vi "Update_Data.vi"(8 "error in (no error)":errorcluster caption="entrée d'erreur (pas d'erreur)", 11 "Firebase Benches en entrée":refnum<class "Firebase Benches.lvclass">) -> (0 "error out":errorcluster caption="sortie d'erreur", 3 "Firebase Benches en sortie":refnum<class "Firebase Benches.lvclass">)   [LabVIEW 2020, in "Library Instrument & Equipement.lvlib" / "Library FireBase.lvlib" / "Firebase Benches.lvclass"]
doc: "Create New document\nPlease initialise the following values\n - Name BDD\n - Document\n - API Key"
uses:
  Firebase Benches.lvclass
  C:/Users/ngarcin/OneDrive - Altyor/Standard TB/Class/Firebase/Source/Firebase Driver/Firebase Driver.lvclass
  Firebase Benches.lvclass/Firebase Benches.ctl
  Firebase Altyor/Firebase Altyor.lvclass
  Firebase Driver/Firebase Driver.lvclass
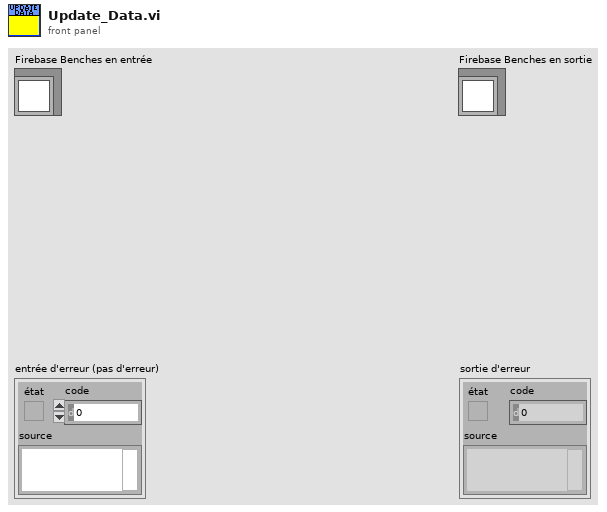
[diagram p1: front panel]
types:
  T1 = cluster{"fields":cluster{"Result":cluster{"booleanValue":bool}, "CreationDate":cluster{"timestampValue":string}, "Batch":cluster{"stringValue":string}, "SerialNumber":cluster{"stringValue":string}, "EndOfProduction":cluster{"timestampValue":string}, "FW_Version":cluster{"mapValue":cluster{"fields":cluster{"Bootloader":cluster{"mapValue":cluster{"fields":cluster{"File_Name":cluster{"stringValue":string}, "Version":cluster{"mapValue":cluster{"fields":cluster{"Major":cluster{"stringValue":string}, "Minor":cluster{"stringValue":string}}}}, "Checksum":cluster{"stringValue":string}}}}, "SoftDevice":cluster{"mapValue":cluster{"fields":cluster{"File_Name":cluster{"stringValue":string}, "Version":cluster{"mapValue":cluster{"fields":cluster{"Major":cluster{"stringValue":string}, "Minor":cluster{"stringValue":string}}}}, "Checksum":cluster{"stringValue":string}}}}, "DFU":cluster{"mapValue":cluster{"fields":cluster{"File_Name":cluster{"stringValue":string}, "Version":cluster{"mapValue":cluster{"fields":cluster{"Major":cluster{"stringValue":string}, "Minor":cluster{"stringValue":string}}}}, "Checksum":cluster{"stringValue":string}}}}}}}, "PartNumber":cluster{"stringValue":string}, "OrderNumber":cluster{"stringValue":string}, "Operator":cluster{"stringValue":string}}}
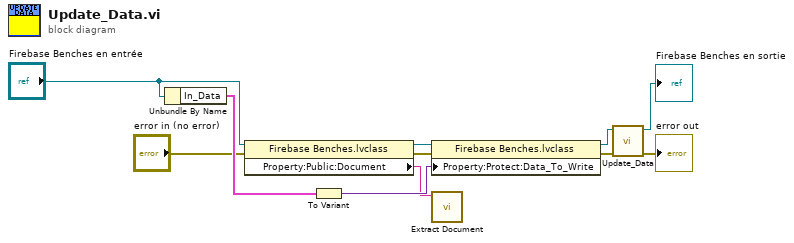
[diagram p0: block diagram]
diagram:
  n1 = Unbundle By Name("Firebase Benches en entrée") -> ("In_Data"=w9:T1)
  n2 = property class="Firebase Benches.lvclass"(reference="Firebase Benches en entrée", error in="error in (no error)") -> (reference out=w5:refnum<class "Firebase Benches.lvclass">, error out=w6:errorcluster, "Property:Public:Document"=w7:string)
  n3 = To Variant(anything=w9) -> (Variant=w8:variant)
  n4 = property class="Firebase Benches.lvclass"(reference=w5, error in=w6, "Property:Protect:Data_To_Write"=w8) -> (reference out=w1:refnum<class "Firebase Benches.lvclass">, error out=w4:errorcluster)
  n5 = call "Extract Document.vi"("Name"=w7) -> ()  [unwired: 9 in, 2 out]
  n6 = call-parent "Update_Data.vi"("error in (no error)"=w4, "Firebase Altyor en entrée"=w1) -> ("error out"=→"error out":errorcluster, "Firebase Altyor en sortie"=→"Firebase Benches en sortie":refnum<class "Firebase Benches.lvclass">)  [unwired: 8 in]
